vi "Twist-Handle Values.vi"() -> (0 "Twist-Handle":T1)   [LabVIEW 2014]
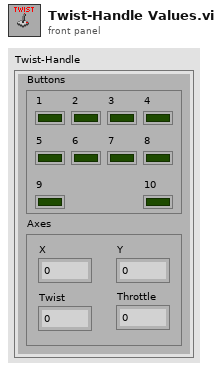
[diagram p1: front panel]
types:
  T1 = cluster{"Buttons":cluster{"1":bool, "2":bool, "3":bool, "4":bool, "5":bool, "6":bool, "7":bool, "8":bool, "9":bool, "10":bool}, "Axes":cluster{"X":dbl, "Y":dbl, "Twist":dbl, "Throttle":dbl}}
  T2 = cluster{"Boolean":bool, "Boolean":bool, "Boolean":bool, "Boolean":bool, "Boolean":bool, "Boolean":bool, "Boolean":bool, "Boolean":bool, "Boolean":bool, "Boolean":bool}
  T3 = cluster{"Numeric":dbl, "Numeric":dbl, "Numeric":dbl, "Numeric":dbl}
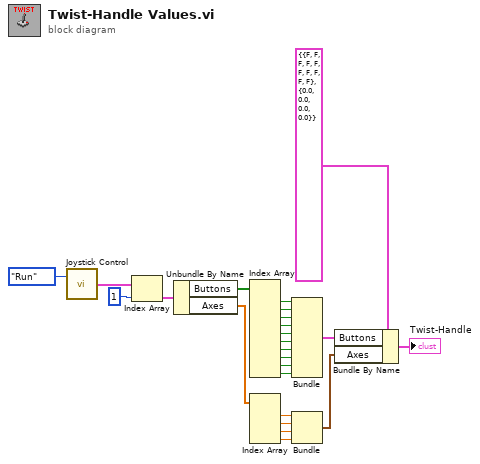
[diagram p0: block diagram]
diagram:
  n1 = call "Joystick Control.vi"("Mode"=enum8{"Start", "Run", "Finish"}."Run") -> ("Joysticks"=w23:cluster{"Buttons":bool[], "Axes":dbl[]}[])  [unwired: 1 in]
  n2 = Index Array(array=w23, index=1) -> (element=w22:cluster{"Buttons":bool[], "Axes":dbl[]})
  n3 = Unbundle By Name(w22) -> ("Buttons"=w21:bool[], "Axes"=w10:dbl[])
  n4 = Index Array(array=w21) -> (element #1=w19:bool, element #2=w20:bool, element #3=w11:bool, element #4=w12:bool, element #5=w13:bool, element #6=w14:bool, element #7=w15:bool, element #8=w16:bool, element #9=w17:bool, element #10=w18:bool)  [unwired: 10 in]
  n5 = Index Array(array=w10) -> (element #1=w8:dbl, element #2=w9:dbl, element #3=w6:dbl, element #4=w7:dbl)  [unwired: 4 in]
  n6 = Bundle("Boolean"=w19, "Boolean"=w20, "Boolean"=w11, "Boolean"=w12, "Boolean"=w13, "Boolean"=w14, "Boolean"=w15, "Boolean"=w16, "Boolean"=w17, "Boolean"=w18) -> (w5:T2)  [unwired: 1 in]
  n7 = Bundle("Numeric"=w8, "Numeric"=w9, "Numeric"=w6, "Numeric"=w7) -> (w4:T3)  [unwired: 1 in]
  n8 = Bundle By Name(cluster=T1 {"Buttons"={"1"=FALSE, "2"=FALSE, "3"=FALSE, "4"=FALSE, "5"=FALSE, "6"=FALSE, "7"=FALSE, "8"=FALSE, "9"=FALSE, "10"=FALSE}, "Axes"={"X"=0.0, "Y"=0.0, "Twist"=0.0, "Throttle"=0.0}} ("Twist-Handle"), "Buttons"=w5, "Axes"=w4) -> (→"Twist-Handle":T1)
